vi "AgNA_Initialize.vi"(8 "error in (no error)":errorcluster {"code" format="%.0x"}, 9 "reset device (Off)":bool, 10 "id query (Off)":bool, 11 "resource name":refnum<k15> caption="resource string") -> (0 "error out":errorcluster {"code" format="%.0x"}, 3 "instrument handle out":refnum<k15>)   [LabVIEW 2015]
uses:
  <instrlib>/Agilent NA/Agilent NA.lvlib
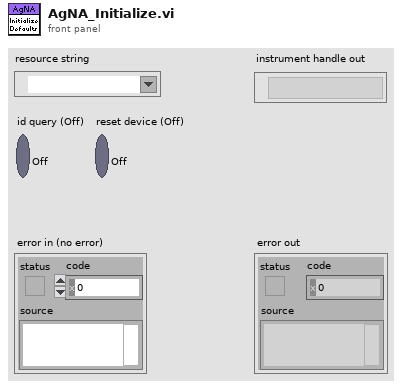
[diagram p1: front panel]
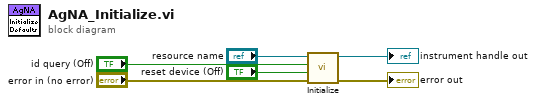
[diagram p0: block diagram]
diagram:
  n1 = call <instrlib>:"Initialize.vi"("error in (no error)"="error in (no error)", "reset device (Off)"="reset device (Off)", "id query (Off)"="id query (Off)", "resource name"="resource name") -> ("error out"=→"error out":errorcluster, "instrument handle out"=→"instrument handle out":refnum<k15>)  [unwired: 6 in]
